vi "Intan_UpdateMarkers_64chan.vi"(0 "ChanSelectMode":u16, 1 "Picture In":picture, 2 "Display Chans":i32[](listbox)=[1, 4, 13, 14, 15, 16, 17, 22], 3 "plot bounds":T1, 4 "YtxtLabelsAll":string[](array[string])) -> (5 "Picture Out":picture, 6 "update labels":bool)   [LabVIEW 2015]
uses:
  <vilib>/Utility/miscctls.llb/LVRectTypeDef.ctl
panel:
  out "Picture":picture
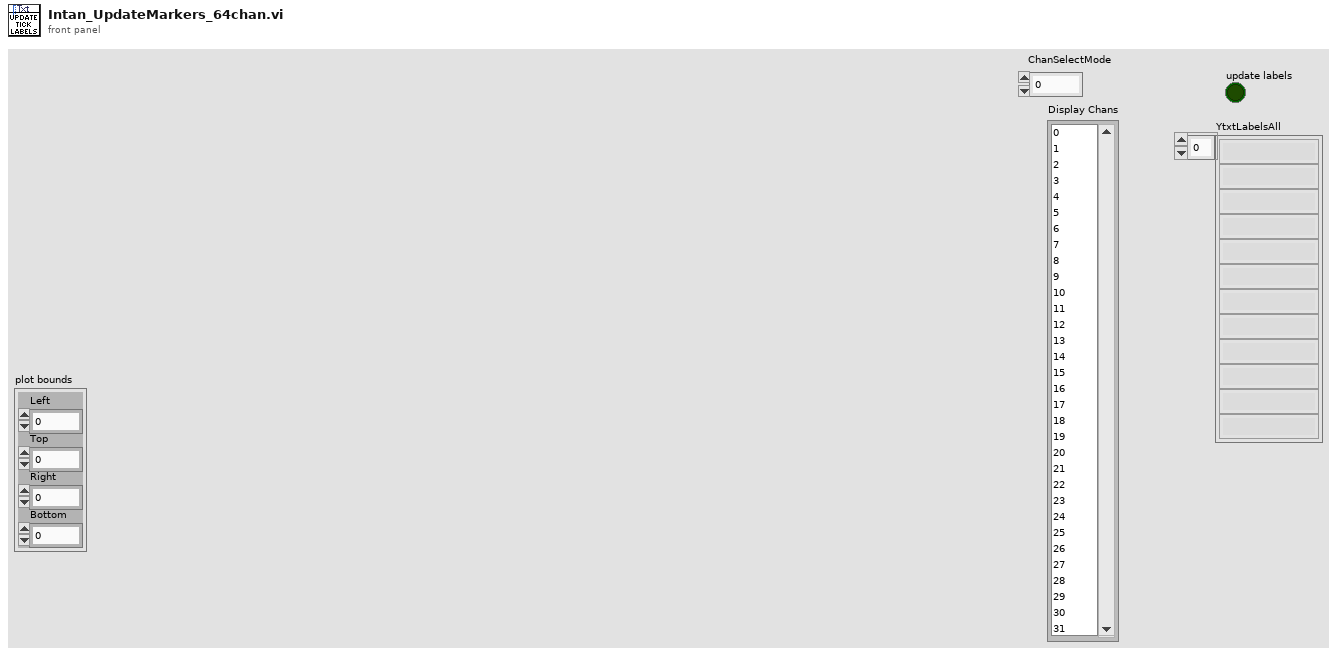
[diagram p1: front panel]
types:
  T1 = typedef "LVRectTypeDef.ctl" = cluster{"Left":i16, "Top":i16, "Right":i16, "Bottom":i16}
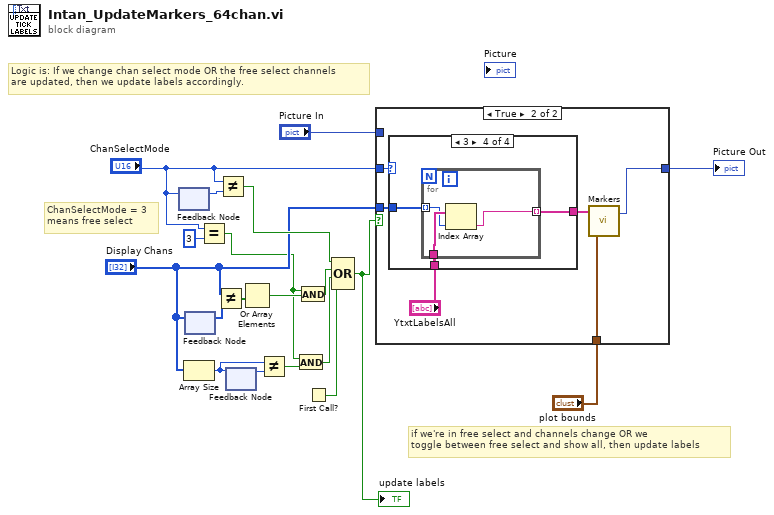
[diagram p0: block diagram]
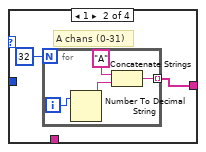
[diagram p4: hidden frame]
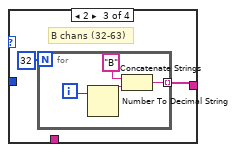
[diagram p5: hidden frame]
diagram:
  # "Logic is: If we change chan select mode OR the free select channels \nare updated, then we update labels accordingly."
  # "ChanSelectMode = 3\nmeans free select"
  # "if we're in free select and channels change OR we\ntoggle between free select and show all, then update labels"
  n1 = feedback #1() -> (w14:u16)  [unwired: 1 in]
  n2 = feedback-in #1("ChanSelectMode") -> ()
  n3 = Array Size(array="Display Chans") -> (size(s)=w13:i32)
  n4 = feedback #2() -> (w18:i32[])  [unwired: 1 in]
  n5 = feedback-in #2("Display Chans") -> ()
  n6 = Equal?(x="ChanSelectMode", y=u16 3) -> (x = y?=w1:bool)
  n7 = Not Equal?(x="Display Chans", y=w18) -> (x != y?=w17:bool[])
  n8 = Not Equal?(x="ChanSelectMode", y=w14) -> (x != y?=w15:bool)
  n9 = feedback #3() -> (w12:i32)  [unwired: 1 in]
  n10 = feedback-in #3(w13) -> ()
  n11 = Or Array Elements(Boolean array=w17) -> (logical OR=w19:bool)
  n12 = Not Equal?(x=w13, y=w12) -> (x != y?=w11:bool)
  n13 = And(x=w1, y=w11) -> (x .and. y?=w10:bool)
  n14 = And(x=w1, y=w19) -> (x .and. y?=w16:bool)
  n15 = First Call?() -> (First Call?: T/F=w9:bool)
  n16 = Compound Arithmetic op=OR(w15, w16, w10, w9) -> (w7:bool)
  "update labels" <- w7
  n17 = case shown="True" w7 {
    tunnel: "ChanSelectMode" -> [_ w25]
    tunnel: "Display Chans" -> [_ w24]
    tunnel: "plot bounds" -> [_ w23]
    tunnel: [w20 w22] -> w5
    tunnel: "Picture In" -> [w20 _]
    frame False {
    }
    frame True {
      n18 = case shown="3" w25 {
        tunnel: w24 -> [_ _ _ w42]
        tunnel: [w27 w29 w34 w41] -> w26
        tunnel: "YtxtLabelsAll" -> [w27 _ _ w40]
        frame 0, Default {
          # "not free select = \n    show all chans"
        }
        frame 1 {
          # "A chans (0-31)"
          n19 = for {
            N: 32 -> [_]
            tunnel: [w31] -> w29 mode=indexing
            i -> [w30]
            n20 = Number To Decimal String(number=w30) -> (decimal integer string=w33:string)  [unwired: 1 in]
            n21 = Concatenate Strings("A" ("string"), w33) -> (w31:string)
          }
        }
        frame 2 {
          # "B chans (32-63)"
          n22 = for {
            N: 32 -> [_]
            tunnel: [w37] -> w34 mode=indexing
            i -> [w36]
            n23 = Number To Decimal String(number=w36) -> (decimal integer string=w39:string)  [unwired: 1 in]
            n24 = Concatenate Strings("B" ("string"), w39) -> (w37:string)
          }
        }
        frame 3 {
          n25 = for {
            tunnel: w42 -> [w44] mode=indexing
            tunnel: [w43] -> w41 mode=indexing
            tunnel: w40 -> [w45]
            n26 = Index Array(array=w45, index=w44) -> (element=w43:string)
          }
        }
      }
      n27 = call "Markers.vi"("plot bounds"=w23, "Array"=w26) -> ("Picture"=w22:picture)  [unwired: 1 out]
    }
  }
  "Picture Out" <- w5
